vi "rethinkdb_initialize.vi"(6 "ms timeout (10000)":i32=10000, 8 "error in (no error)":errorcluster, 9 "version (10=v1_0)":u8=10, 10 "port (28015)":u16=28015, 11 "host (\"localhost\")":string="localhost") -> (0 "error out":errorcluster, 2 "handshake":T1, 3 "rethinkdb":refnum<k5>)   [LabVIEW 2017]
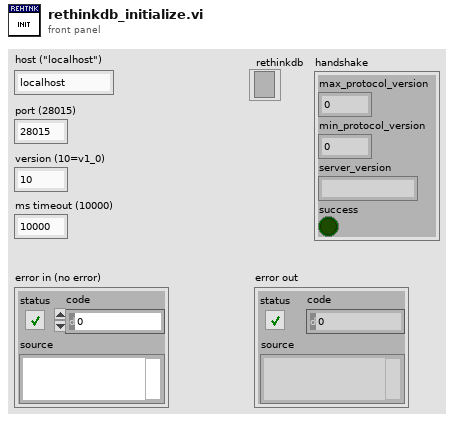
[diagram p1: front panel]
types:
  T1 = cluster{"max_protocol_version":u64, "min_protocol_version":u64, "server_version":string, "success":bool}
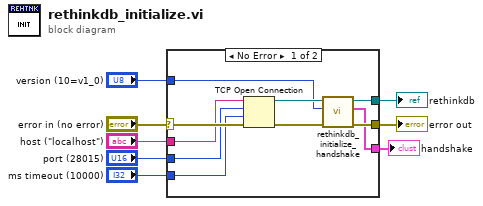
[diagram p0: block diagram]
diagram:
  n1 = case shown="No Error" "error in (no error)" {
    selector: "error in (no error)" -> [w18 w19]
    tunnel: "host (\"localhost\")" -> [w17 _]
    tunnel: "port (28015)" -> [w16 _]
    tunnel: "ms timeout (10000)" -> [w15 _]
    tunnel: [w13 w19] -> w4
    tunnel: [w11 _] -> w3
    tunnel: "version (10=v1_0)" -> [w10 _]
    tunnel: [w9 _] -> w1
    frame No Error {
      n2 = TCP Open Connection(address=w17, remote port or service name=w16, timeout ms (60000)=w15, error in (no error)=w18) -> (connection ID=w12:refnum<k5>, error out=w14:errorcluster)  [unwired: 1 in]
      n3 = call "rethinkdb_initialize_handshake.vi"("error in (no error)"=w14, "version (10=v1_0)"=w10, "rethinkdb in"=w12) -> ("error out"=w13:errorcluster, "handshake"=w9:T1, "rethinkdb out"=w11:refnum<k5>)  [unwired: 6 in]
    }
    frame Error {
    }
  }
  "error out" <- w4
  "rethinkdb" <- w3
  "handshake" <- w1
